vi "Choose Search Mode.vi"(9 "Last Cam-Relative Y":dbl, 11 "Last Cam-Relative X":dbl) -> (2 "Search Dir":T1)   [LabVIEW 2013]
uses:
  Camera Search State.ctl
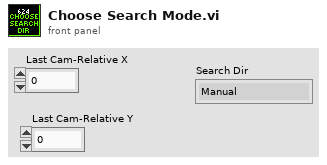
[diagram p1: front panel]
types:
  T1 = typedef "Camera Search State.ctl" = enum16{"Manual", "Search Left", "Search Right", "Target Found", "Disabled", "Search Down", "Search Up"}
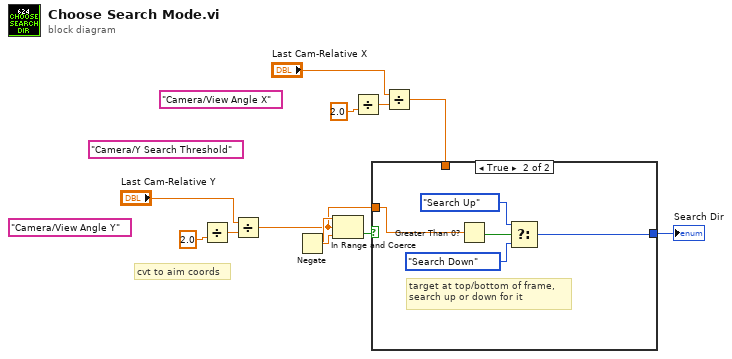
[diagram p0: block diagram]
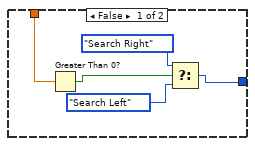
[diagram p2: hidden frame]
diagram:
  w7 = "Camera/Y Search Threshold" ("Name")
  w15 = "Camera/View Angle Y" ("Name")
  w14 = "Camera/View Angle X" ("Name")
  # "cvt to aim coords"
  n1 = Divide(y=2.0) -> (x=w16:dbl, x/y=w9:dbl)
  n2 = Divide(x="Last Cam-Relative Y", y=w9) -> (x/y=w3:dbl)
  n3 = Divide(y=2.0) -> (x=w13:dbl, x/y=w10:dbl)
  n4 = Divide(x="Last Cam-Relative X", y=w10) -> (x/y=w1:dbl)
  n5 = Negate(x=w5) -> (-x=w6:dbl)
  n6 = In Range and Coerce(x=w3, lower limit=w6) -> (upper limit=w5:dbl, In Range?=w4:bool)  [unwired: 1 out]
  n7 = case shown="True" w4 {
    tunnel: w3 -> [_ w27]
    tunnel: [w19 w23] -> w2
    tunnel: w1 -> [w22 _]
    frame False {
      n8 = Greater Than 0?(x=w22) -> (x > 0?=w20:bool)
      n9 = Select(t=Camera_Search_State."Search Right" ("Enum"), s=w20, f=Camera_Search_State."Search Left" ("Enum")) -> (s? t:f=w19:T1)
    }
    frame True {
      # "target at top/bottom of frame,\nsearch up or down for it"
      n10 = Greater Than 0?(x=w27) -> (x > 0?=w26:bool)
      n11 = Select(t=Camera_Search_State."Search Up" ("Enum"), s=w26, f=Camera_Search_State."Search Down" ("Enum")) -> (s? t:f=w23:T1)
    }
  }
  "Search Dir" <- w2
